vi "Host Send Command.vi"() -> ()   [LabVIEW 2026]
uses:
  RT Commands.ctl
  RT States.ctl
  Game Settings.ctl
panel:
  in  "Game Settings":T1
  out "RT2HState":T2=enum."Configuring"
  in  "H2RTCommand":T3=enum."Commit Settings"
  in  "stop":bool
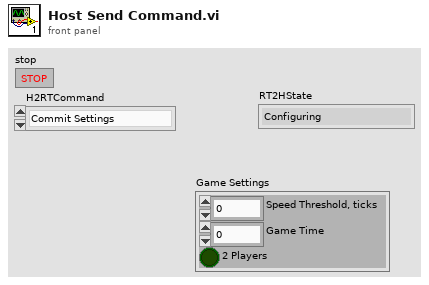
[diagram p1: front panel]
types:
  T1 = typedef "Game Settings.ctl" = cluster{"Speed Threshold, ticks":u64, "Game Time":u32, "2 Players":bool}
  T2 = typedef "RT States.ctl" = enum16{"Idle", "Configuring", "1Player", "2Player", "Display Winner"}
  T3 = typedef "RT Commands.ctl" = enum16{"<null>", "End Idle", "Reset", "Commit Settings", "Commit Host Settings"}
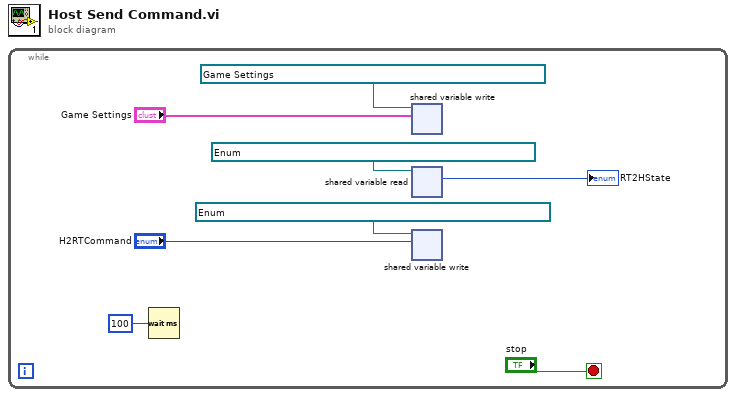
[diagram p0: block diagram]
diagram:
  n1 = while {
    stop <- "stop" stop-if-true
    w3 = refnum<k21> "ni.var.psp://SpeedOfVIght/RT ShardVariables/H2RTCommand" items=["<null>", "End Idle", "Reset", "Commit Settings", "Commit Host Settings"] ("shared variable refnum in")
    w2 = refnum<k21> "ni.var.psp://SpeedOfVIght/RT ShardVariables/RT2HState" items=["Idle", "Configuring", "1Player", "2Player", "Display Winner"] ("shared variable refnum in")
    n2 = Wait (ms)(milliseconds to wait=u32 100) -> ()  [unwired: 1 out]
    n3 = shared-variable-write(refnum<k21> "ni.var.psp://SpeedOfVIght/RT ShardVariables/Game Settings" ("shared variable refnum in"), "Game Settings") -> ()  [unwired: 1 in, 2 out]
    n4 = shared-variable-read(w2) -> (→"RT2HState":T2)  [unwired: 1 in, 2 out]
    n5 = shared-variable-write(w3, "H2RTCommand") -> ()  [unwired: 1 in, 2 out]
  }
